vi "Verify Module Positions.vi"(8 "error in":errorcluster, 10 "Module Positions In":T1[](array[typedef])) -> (0 "error out":errorcluster, 2 "All Good":bool)   [LabVIEW 2017]
uses:
  Procedure Classes/Potting Procedure/Type Definitions/Inspect Modules - Module.ctl
  Shared Components/Vec3d Class/Vec3d Class.lvclass
  Shared Components/Utils/Type Definitions/Multi-Fiducial Image.ctl
  Shared Components/Utils/Type Definitions/Physical Image.ctl
  <vilib>/vision/Image Controls.llb/IMAQ Image.ctl
  Shared Components/Utils/Type Definitions/Fiducial with Source.ctl
  Shared Components/Utils/Type Definitions/Fiducial Image.ctl
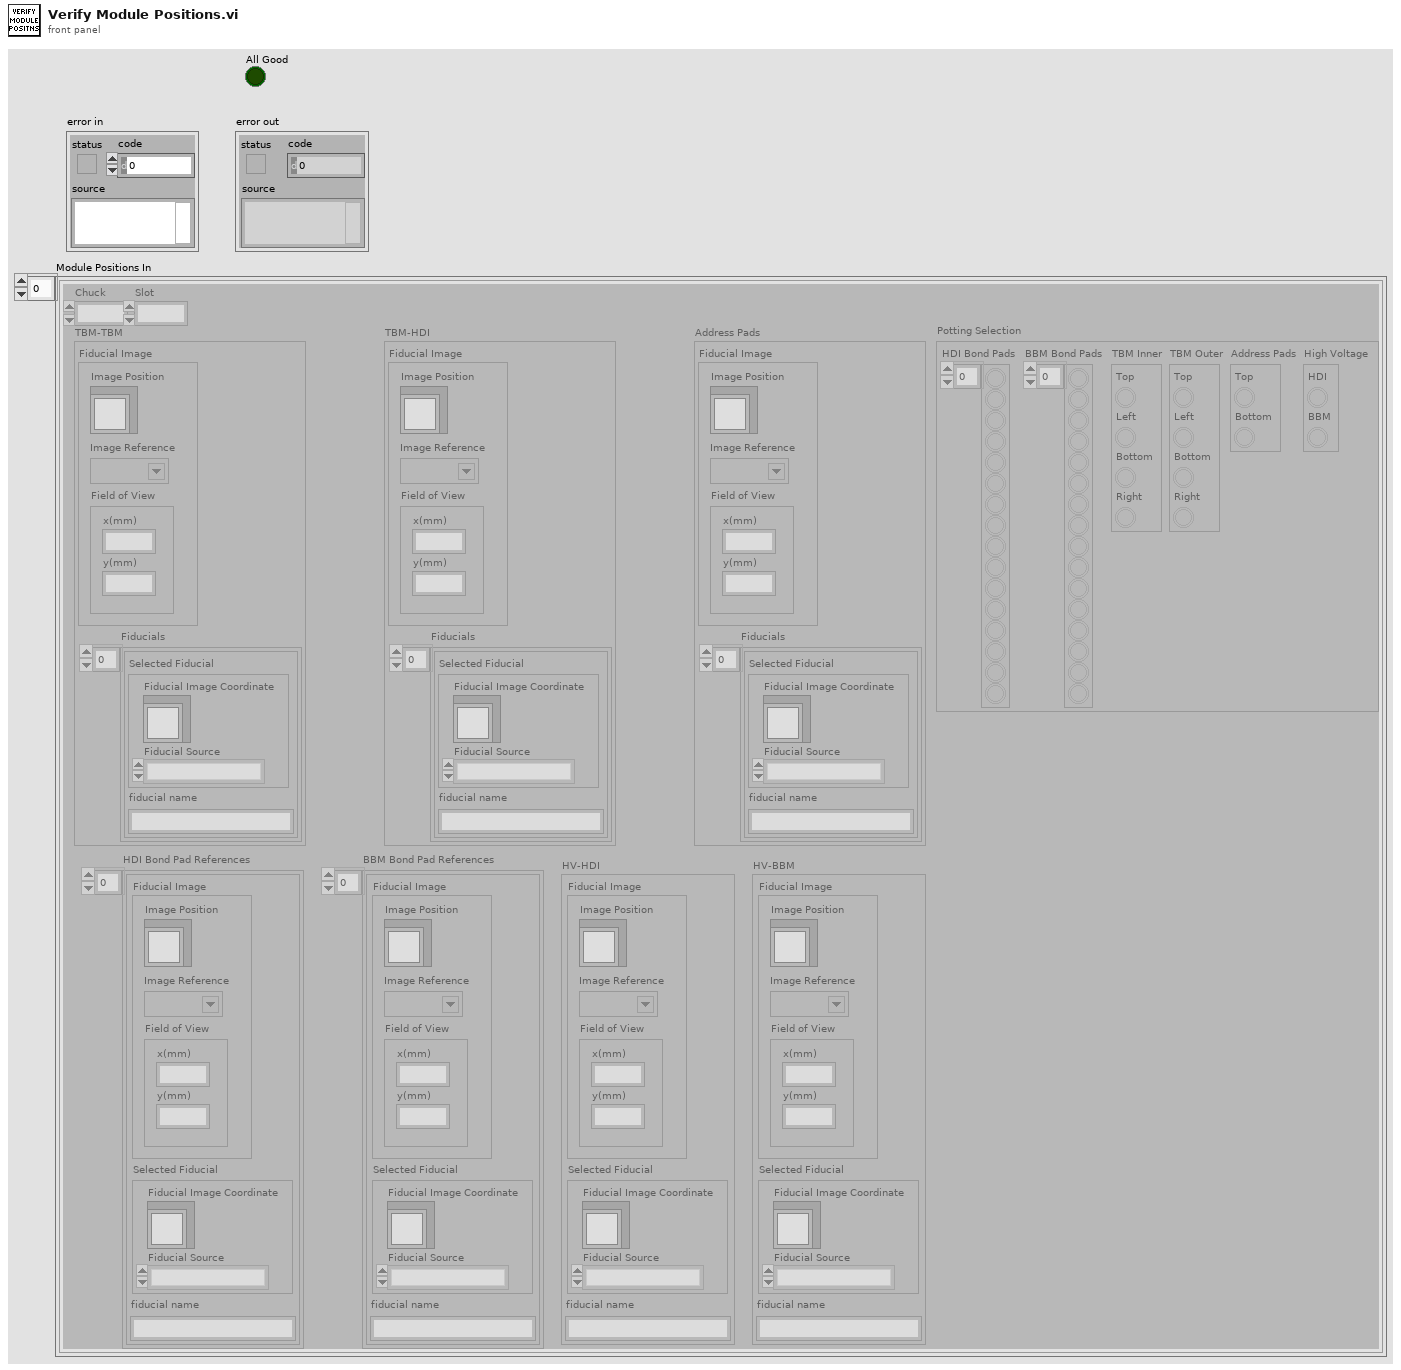
[diagram p1: front panel]
types:
  T1 = typedef "Inspect Modules - Module.ctl" = cluster{"TBM-TBM":T2, "TBM-HDI":T2, "Address Pads":T2, "HDI Bond Pad References":T6[], "BBM Bond Pad References":T6[], "HV-HDI":T6, "HV-BBM":T6, "Chuck":i32, "Slot":i32, "Potting Selection":cluster{"HDI Bond Pads":bool[], "BBM Bond Pads":bool[], "TBM Inner":cluster{"Top":bool, "Left":bool, "Bottom":bool, "Right":bool}, "TBM Outer":cluster{"Top":bool, "Left":bool, "Bottom":bool, "Right":bool}, "Address Pads":cluster{"Top":bool, "Bottom":bool}, "High Voltage":cluster{"HDI":bool, "BBM":bool}}}
  T2 = typedef "Multi-Fiducial Image.ctl" = cluster{"Fiducial Image":T3, "Fiducials":cluster{"Selected Fiducial":T5, "fiducial name":string}[]}
  T3 = typedef "Physical Image.ctl" = cluster{"Image Position":refnum<class "Vec3d Class.lvclass">, "Image Reference":T4, "Field of View":cluster{"x(mm)":dbl, "y(mm)":dbl}}
  T4 = typedef "IMAQ Image.ctl" = refnum<image>
  T5 = typedef "Fiducial with Source.ctl" = cluster{"Fiducial Image Coordinate":refnum<class "Vec3d Class.lvclass">, "Fiducial Source":enum16{"Pattern Recognition", "User", "Error", "Default"}}
  T6 = typedef "Fiducial Image.ctl" = cluster{"Fiducial Image":T3, "Selected Fiducial":T5, "fiducial name":string}
  T7 = enum16{"Pattern Recognition", "User", "Error", "Default"}
  T8 = cluster{"Selected Fiducial":T5, "fiducial name":string}[]
  T9 = enum16{"Pattern Recognition", "User", "Error", "Default"}[]
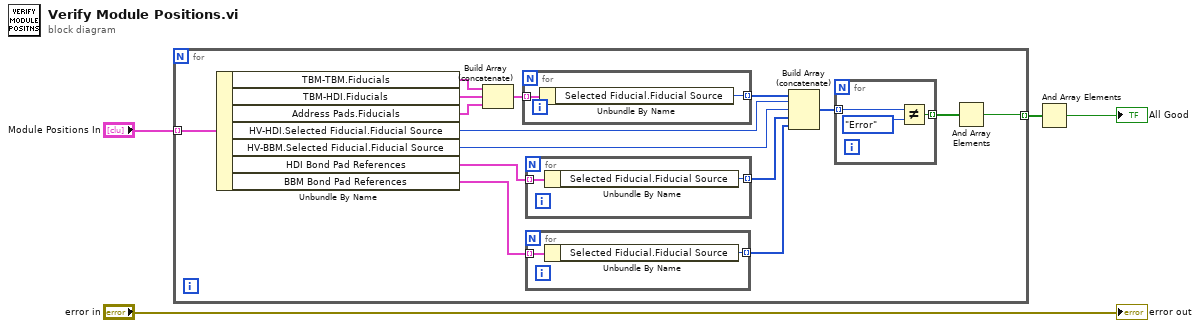
[diagram p0: block diagram]
diagram:
  n1 = for {
    tunnel: "Module Positions In" -> [w19] mode=indexing
    tunnel: [w5] -> w3 mode=indexing
    n2 = Unbundle By Name(w19) -> ("TBM-TBM.Fiducials"=w18:T8, "TBM-HDI.Fiducials"=w17:T8, "Address Pads.Fiducials"=w16:T8, "HV-HDI.Selected Fiducial.Fiducial Source"=w11:T7, "HV-BBM.Selected Fiducial.Fiducial Source"=w10:T7, "HDI Bond Pad References"=w15:T6[], "BBM Bond Pad References"=w14:T6[])
    n3 = Build Array (concatenate)(w18, w17, w16) -> (w13:T8)
    n4 = for {
      tunnel: w13 -> [w24] mode=indexing
      tunnel: [w23] -> w12 mode=indexing
      n5 = Unbundle By Name(w24) -> ("Selected Fiducial.Fiducial Source"=w23:T7)
    }
    n6 = for {
      tunnel: w15 -> [w28] mode=indexing
      tunnel: [w27] -> w9 mode=indexing
      n7 = Unbundle By Name(w28) -> ("Selected Fiducial.Fiducial Source"=w27:T7)
    }
    n8 = for {
      tunnel: w14 -> [w26] mode=indexing
      tunnel: [w25] -> w8 mode=indexing
      n9 = Unbundle By Name(w26) -> ("Selected Fiducial.Fiducial Source"=w25:T7)
    }
    n10 = Build Array (concatenate)(w12, w11, w10, w9, w8) -> (w7:T9)
    n11 = for {
      tunnel: w7 -> [w22] mode=indexing
      tunnel: [w20] -> w6 mode=indexing
      n12 = Not Equal?(x=w22, y=T7."Error") -> (x != y?=w20:bool)
    }
    n13 = And Array Elements(Boolean array=w6) -> (logical AND=w5:bool)
  }
  n14 = And Array Elements(Boolean array=w3) -> (logical AND=→"All Good":bool)
  "error out" <- "error in"
